vi "Blocker Auto.vi"(1 "Run?":bool) -> (0 "Done?":bool)   [LabVIEW 2013]
uses:
  Globals/Useful Values.vi
  <vilib>/addons/control/pid/NI_PID_pid.lvlib
  <vilib>/addons/control/pid/pid.llb/PID (DBL).vi
panel:
  in  "Gain":dbl
  in  "In":dbl
  out "Left Setpoint":dbl
  out "Right Setpoint":dbl
  out "Right Output":dbl
  out "Left Output":dbl
  in  "PID gains":T1 {"derivative time (Td, min)" format="%.3f"; "integral time (Ti, min)" format="%.3f"; "proportional gain (Kc)" format="%.3f"}
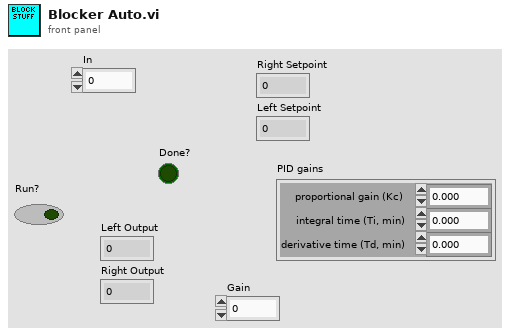
[diagram p1: front panel]
types:
  T1 = cluster{"proportional gain (Kc)":dbl, "integral time (Ti, min)":dbl, "derivative time (Td, min)":dbl}
  T2 = typedef "WPI_AnalogChannelDevRef.ctl" = cluster{"DevStatus":errorcluster, "Analog Module":T3, "Analog Channel":T4}
  T3 = typedef "FPGA_TypedefAnalogModule.ctl" = enum16{"Analog Module 1", "Analog Module 2"}
  T4 = typedef "FPGA_AIChannel.ctl" = enum8{"AI 1", "AI 2", "AI 3", "AI 4", "AI 5", "AI 6", "AI 7", "AI 8", "Invalid"}
  T5 = typedef "WPI_EncoderDevRef.ctl" = cluster{"DevStatus":errorcluster, "EncoderIndex":T6, "CounterIndex":T7, "DistancePerCount":dbl, "Decoding Type":T8}
  T6 = typedef "FPGA_EncoderIdx.ctl" = enum8{"Enc 0", "Enc 1", "Enc 2", "Enc 3", "Invalid"}
  T7 = typedef "FPGA_CounterCtrSystemIndex.ctl" = enum8{"Ctr 0", "Ctr 1", "Ctr 2", "Ctr 3", "Ctr 4", "Ctr 5", "Ctr 6", "Ctr 7", "Invalid"}
  T8 = typedef "WPI_EncoderType.ctl" = enum16{"1x", "2x", "4x"}
  T9 = typedef "WPI_MotorControlDeviceRef.ctl" = cluster{"DeviceStatus":errorcluster, "Type":enum16{"PWM", "CAN"}, "PWM":cluster{"Digital Module":T10, "PWM Channel":T11, "DeadBand":T12}, "CAN":cluster{"Device Number":u8, "Control Mode":T13, "Semaphore":T14, "Max Vout":dbl}, "Invert":bool, "TransformRef":T15, "InvTransformRef":T15}
  T10 = typedef "FPGA_TypedefDigitalModule.ctl" = enum16{"Digital Module 1", "Digital Module 2"}
  T11 = typedef "FPGA_DIOPWMChannel.ctl" = enum8{"PWM 1", "PWM 2", "PWM 3", "PWM 4", "PWM 5", "PWM 6", "PWM 7", "PWM 8", "PWM 9", "PWM 10", "Invalid"}
  T12 = typedef "WPI_PWMDeadband.ctl" = cluster{"Name":string, "maxPositivePwm":i32, "minPositivePwm":i32, "centerPwm":i32, "maxNegativePwm":i32, "minNegativePwm":i32, "angularRange":u16}
  T13 = typedef "WPI_CANJaguar_ControlMode.ctl" = enum8{"Percent VBus", "Current", "Speed", "Position", "Voltage"}
  T14 = typedef "Semaphore RefNum" = refnum<k1>
  T15 = typedef "WPI_PWMTransform_ConPane.ctl" = refnum<vi>
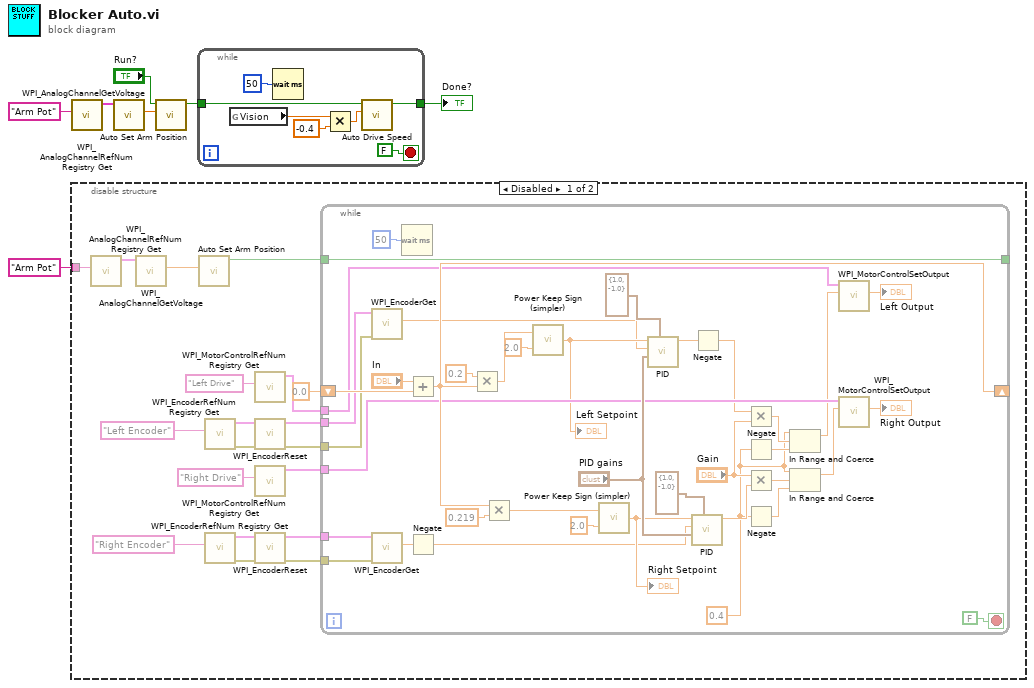
[diagram p0: block diagram]
diagram:
  n1 = call <vilib>:"WPI_AnalogChannelRefNum Registry Get.vi"("refnum name"="Arm Pot") -> ("AIDeviceRef"=w6:T2)  [unwired: 9 in, 1 out]
  n2 = disable-structure shown="Disabled" {
    disable-tunnel: "Arm Pot" ("refnum name") -> [w26 _]
    frame Disabled {
      n3 = call <vilib>:"WPI_AnalogChannelRefNum Registry Get.vi"("refnum name"=w26) -> ("AIDeviceRef"=w27:T2)  [unwired: 9 in, 1 out]
      n4 = call <vilib>:"WPI_AnalogChannelGetVoltage.vi"("AIDeviceRef"=w27) -> ("Voltage"=w25:dbl)  [unwired: 8 in, 2 out]
      n5 = call "Auto Set Arm Position.vi"("Arm Position"=w25) -> ("Done"=w24:bool)  [unwired: 10 in]
      n6 = call <vilib>:"WPI_EncoderRefNum Registry Get.vi"("refnum name"="Left Encoder") -> ("error out"=w21:errorcluster, "EncoderDevRef"=w20:T5)  [unwired: 9 in]
      n7 = call <vilib>:"WPI_EncoderRefNum Registry Get.vi"("refnum name"="Right Encoder") -> ("error out"=w18:errorcluster, "EncoderDevRef"=w19:T5)  [unwired: 9 in]
      n8 = call <vilib>:"WPI_MotorControlRefNum Registry Get.vi"("refnum name"="Left Drive") -> ("MotorControlDevRef"=w11:T9)  [unwired: 9 in, 1 out]
      n9 = call <vilib>:"WPI_EncoderReset.vi"("error in (no error)"=w21, "EncoderDevRef"=w20) -> ("error out"=w15:errorcluster, "EncoderDevRef"=w14:T5)  [unwired: 8 in]
      n10 = call <vilib>:"WPI_MotorControlRefNum Registry Get.vi"("refnum name"="Right Drive") -> ("MotorControlDevRef"=w8:T9)  [unwired: 9 in, 1 out]
      n11 = call <vilib>:"WPI_EncoderReset.vi"("error in (no error)"=w18, "EncoderDevRef"=w19) -> ("error out"=w16:errorcluster, "EncoderDevRef"=w17:T5)  [unwired: 8 in]
      n12 = while {
        tunnel: w24 -> [w65]
        tunnel: [w65] -> w23
        shift-right: [w62] -> _
        shift-left: 0.0 -> [w63]
        tunnel: w17 -> [w57]
        tunnel: w16 -> [w56]
        tunnel: w15 -> [w55]
        tunnel: w14 -> [w54]
        tunnel: w11 -> [w52]
        tunnel: w8 -> [w51]
        stop <- FALSE stop-if-true
        w29 = 0.4 ("upper limit")
        n13 = call <vilib>:"WPI_EncoderGet.vi"("error in (no error)"=w55, "EncoderDevRef"=w54) -> ("Distance"=w43:dbl)  [unwired: 4 in, 5 out]
        n14 = call <vilib>:"WPI_EncoderGet.vi"("error in (no error)"=w56, "EncoderDevRef"=w57) -> ("Distance"=w40:dbl)  [unwired: 4 in, 5 out]
        n15 = Wait (ms)(milliseconds to wait=u32 50) -> ()  [unwired: 1 out]
        n16 = Add(x="In", y=w63) -> (x+y=w62:dbl)
        n17 = Negate(x=w40) -> (-x=w38:dbl)
        n18 = Multiply(x=0.2, y=w62) -> (x*y=w47:dbl)
        n19 = Multiply(x=w62, y=0.219) -> (x*y=w50:dbl)
        n20 = call "Power Keep Sign (simpler).vi"("Power"=2.0, "In"=w47) -> ("Out"=w45:dbl)
        "Left Setpoint" <- w45
        n21 = call "Power Keep Sign (simpler).vi"("Power"=2.0, "In"=w50) -> ("Out"=w49:dbl)
        "Right Setpoint" <- w49
        n22 = call-poly <vilib>:"PID.vi"("output range"=cluster{"output high":dbl, "output low":dbl} {"output high"=1.0, "output low"=-1.0}, "PID gains"="PID gains", "process variable"=w43, "setpoint"=w45) -> ("output"=w42:dbl)  [unwired: 6 in, 1 out]
        n23 = call-poly <vilib>:"PID.vi"("output range"=cluster{"output high":dbl, "output low":dbl} {"output high"=1.0, "output low"=-1.0}, "PID gains"="PID gains", "process variable"=w38, "setpoint"=w49) -> ("output"=w35:dbl)  [unwired: 6 in, 1 out]
        n24 = Negate(x=w42) -> (-x=w36:dbl)
        n25 = Multiply(x=w36, y="Gain") -> (x*y=w34:dbl)
        n26 = Negate(x=w29) -> (-x=w33:dbl)
        n27 = Multiply(x="Gain", y=w35) -> (x*y=w31:dbl)
        n28 = Negate(x=w29) -> (-x=w30:dbl)
        n29 = In Range and Coerce(upper limit=w29, x=w34, lower limit=w33) -> (coerced(x)=w32:dbl)  [unwired: 1 out]
        n30 = In Range and Coerce(upper limit=w29, x=w31, lower limit=w30) -> (coerced(x)=w28:dbl)  [unwired: 1 out]
        n31 = call <vilib>:"WPI_MotorControlSetOutput.vi"("Output"=w32, "MotorControlDevRef"=w52) -> ("Motor Output"=→"Left Output":dbl)  [unwired: 7 in, 2 out]
        n32 = call <vilib>:"WPI_MotorControlSetOutput.vi"("Output"=w28, "MotorControlDevRef"=w51) -> ("Motor Output"=→"Right Output":dbl)  [unwired: 7 in, 2 out]
      }
    }
    frame Enabled {
    }
  }
  n33 = call <vilib>:"WPI_AnalogChannelGetVoltage.vi"("AIDeviceRef"=w6) -> ("Voltage"=w4:dbl)  [unwired: 8 in, 2 out]
  n34 = call "Auto Set Arm Position.vi"("Arm Position"=w4, "Run?"="Run?") -> ("Done"=w2:bool)  [unwired: 9 in]
  n35 = while {
    tunnel: [w69] -> w1
    tunnel: w2 -> [w67]
    stop <- FALSE stop-if-true
    n36 = global read "Useful Values.vi" "Vision"() -> (w71:dbl)
    n37 = Wait (ms)(milliseconds to wait=u32 50) -> ()  [unwired: 1 out]
    n38 = Multiply(x=w71, y=-0.4) -> (x*y=w70:dbl)
    n39 = call "Auto Drive Speed.vi"("Output"=w70, "Run?"=w67) -> ("Done"=w69:bool)  [unwired: 9 in]
  }
  "Done?" <- w1
